vi "read_params.vi"(8 "error in (no error)":errorcluster, 11 "KNeighborsRegressor in":refnum<class "KNeighborsRegressor.lvclass">) -> (0 "error out":errorcluster, 2 "params":T1={"n_neighbors"=5.0, "weights"="uniform", "algorithm"="auto", "leaf_size"=30.0, "p"=2.0, "metric"="minkowski", "n_jobs"=1.0}, 3 "KNeighborsRegressor out":refnum<class "KNeighborsRegressor.lvclass">)   [LabVIEW 2020, in "KNeighborsRegressor.lvclass"]
uses:
  KNeighborsRegressor.lvclass
  Controls/kneighbors_regressor_params.ctl
  KNeighborsRegressor.lvclass/KNeighborsRegressor.ctl
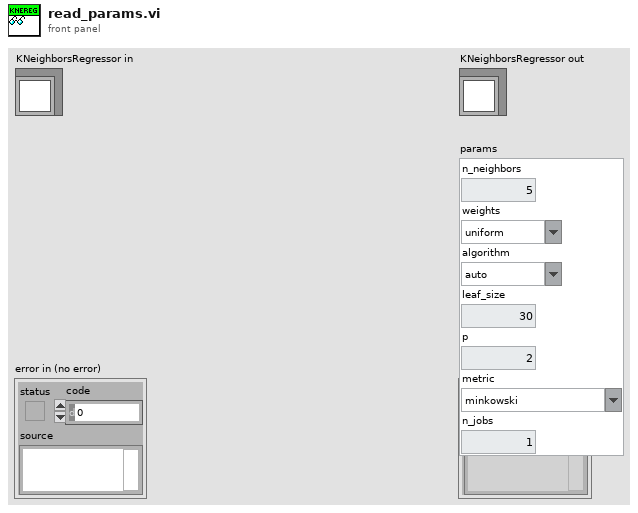
[diagram p1: front panel]
types:
  T1 = typedef "kneighbors_regressor_params.ctl" = cluster{"n_neighbors":dbl, "weights":string, "algorithm":string, "leaf_size":dbl, "p":dbl, "metric":string, "n_jobs":dbl}
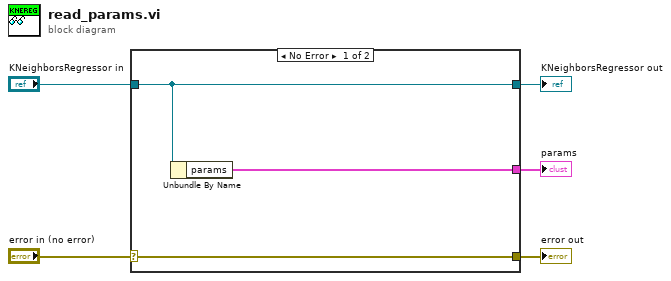
[diagram p0: block diagram]
diagram:
  n1 = case shown="No Error" "error in (no error)" {
    selector: "error in (no error)" -> [w8 w9]
    tunnel: [w8 w9] -> w4
    tunnel: [w7 w10] -> w2
    tunnel: "KNeighborsRegressor in" -> [w7 w10]
    tunnel: [w6 _] -> w1
    frame No Error {
      n2 = Unbundle By Name(w7) -> ("params"=w6:T1)
    }
    frame Error {
    }
  }
  "error out" <- w4
  "KNeighborsRegressor out" <- w2
  "params" <- w1
